vi "RT Driver VI.vi"(7 "Operation":T1, 11 "Device Reference in":T2 format="%.0x") -> (0 "Error Code":i32)   [LabVIEW 2019, in "Telemetry Engine.lvlib"]
uses:
  Telemetry Engine.lvlib
  <vilib>/NI VeriStand/Custom Device API/Custom Device Item Ref.ctl
  <vilib>/NI VeriStand/Custom Device API/Hardware Interface Driver VI Operation.ctl
  Types/Engine State Data.ctl
  Types/Engine Logging Data.ctl
  <vilib>/NI VeriStand/Custom Device API/Block Data Reference.ctl
  <vilib>/NI VeriStand/Custom Device API/Data Reference.ctl
  <vilib>/NI VeriStand/Custom Device API/Global Data Refs.vi
  <vilib>/NI VeriStand/Custom Device API/Custom Device API.lvlib
panel:
  in  "State Data":T3 {"Logging Data"."System Channel Refs" format="%.0x"; "Logging Data"."Block Data Refs"."Data Reference" format="%.0x"}
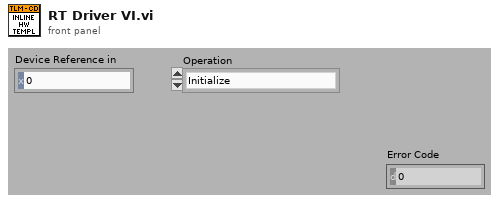
[diagram p1: front panel]
types:
  T1 = typedef "Custom Device API.lvlib/Hardware Interface Driver VI Operation.ctl" = enum16{"Initialize", "Start", "Read Data from HW", "Write Data to HW", "Close"}
  T2 = typedef "Custom Device API.lvlib/Custom Device Item Ref.ctl" = u64
  T3 = typedef "Telemetry Engine.lvlib/Engine State Data.ctl" = cluster{"Data FIFO":refnum<k33>, "Logging Data":T4, "Data FIFO Timeout?":bool, "Data FIFO Timeout Count":dbl, "error":errorcluster}
  T4 = typedef "Telemetry Engine.lvlib/Engine Logging Data.ctl" = cluster{"System Channel Refs":T2[], "Block Data Refs":T5[], "Data Values Array":dbl[], "Data FIFO Timeout Block Ref":i32, "Log File Path":path}
  T5 = typedef "Custom Device API.lvlib/Block Data Reference.ctl" = cluster{"Data Reference":T6, "Offset":u64, "Length":u64}
  T6 = typedef "Custom Device API.lvlib/Data Reference.ctl" = i32
  T7 = cluster{"read mode":enum16{"polling", "blocking"}, "write mode":enum16{"polling", "blocking"}}
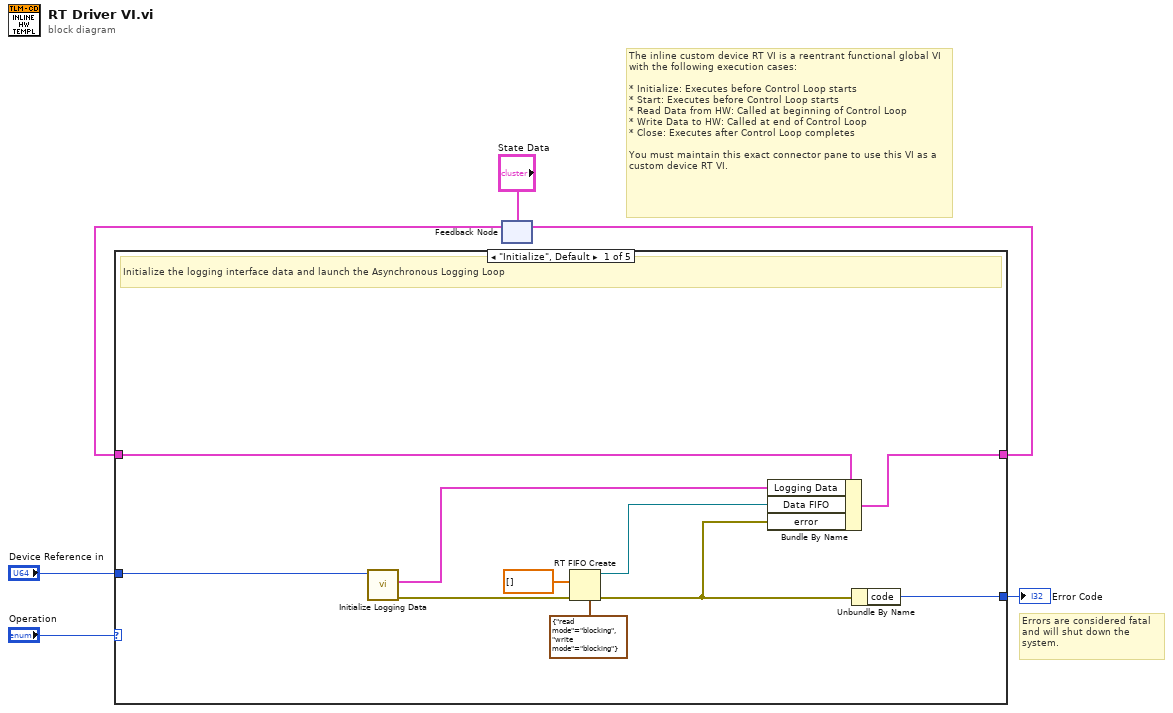
[diagram p0: block diagram]
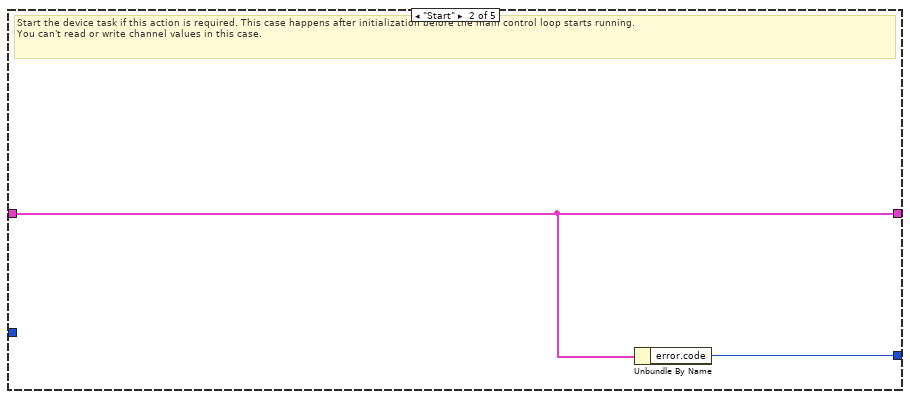
[diagram p2: hidden frame]
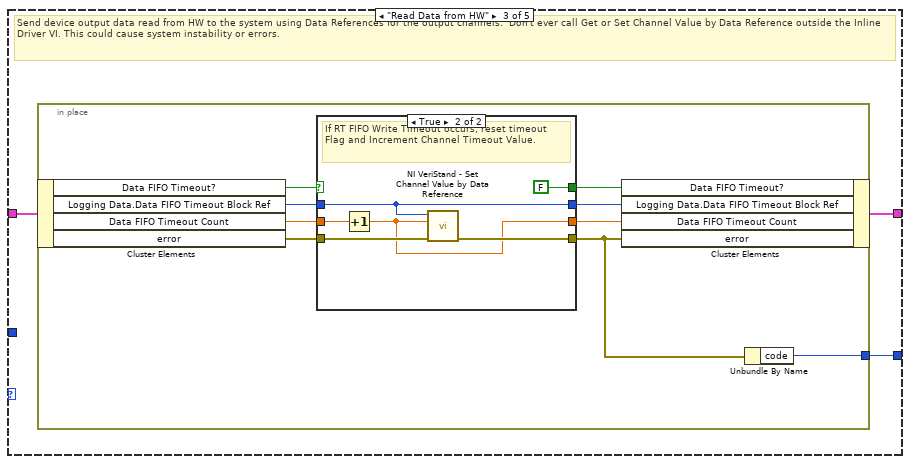
[diagram p3: hidden frame]
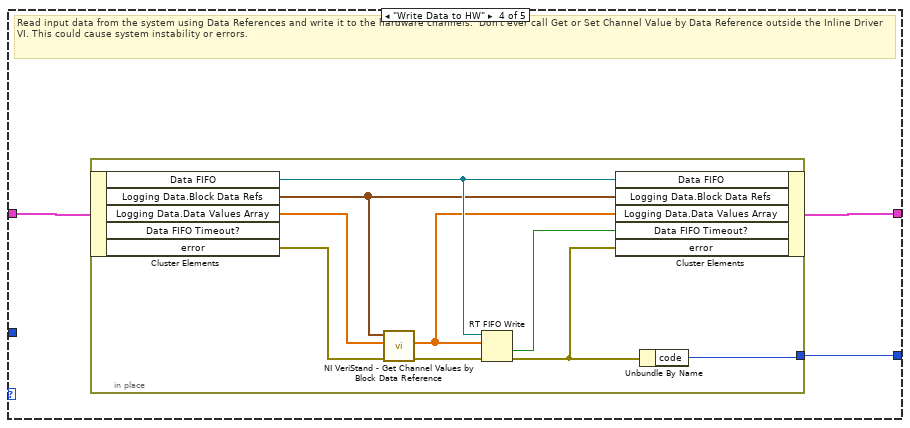
[diagram p5: hidden frame]
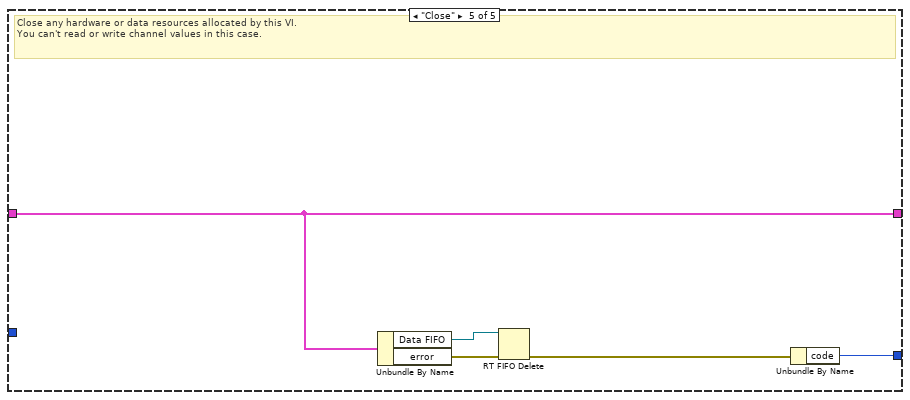
[diagram p6: hidden frame]
diagram:
  # "Errors are considered fatal and will shut down the system."
  # "The inline custom device RT VI is a reentrant functional global VI with the following execution cases:\n\n* Initialize: Executes before Control Loop starts\n* Start: Executes before Control Loop starts\n* Read Data from HW: Called at beginning of Control Loop\n* Write Data to HW: Called at end of Control Loop\n* Close: Executes after Control Loop completes\n\nYou must maintain this exact connector pane to use this VI as a custom device RT VI."
  n1 = feedback #1("State Data") -> (w4:T3)
  n2 = case shown="\"Initialize\", Default" "Operation" {
    tunnel: [w14 w17 w19 w41 w56] -> w5
    tunnel: w4 -> [w13 w17 w20 w42 w56]
    tunnel: "Device Reference in" -> [w9 _ _ _ _]
    tunnel: [w16 w18 w21 w43 w57] -> w2
    frame "Initialize", Default {
      # "Initialize the logging interface data and launch the Asynchronous Logging Loop"
      n3 = call "Initialize Logging Data.vi"("Device Reference in"=w9) -> ("error out"=w7:errorcluster, "Logging Data"=w8:T4)  [unwired: 8 in, 1 out]
      n4 = RT FIFO Create(1:dbl[] [], 3:w7, 7:T7 {"read mode"=enum."blocking", "write mode"=enum."blocking"} ("r/w modes (polling,polling)")) -> (8:w15:refnum<k33>, 11:w12:errorcluster)  [unwired: 5 in, 1 out]
      n5 = Bundle By Name(cluster=w13, "Logging Data"=w8, "Data FIFO"=w15, "error"=w12) -> (w14:T3)
      n6 = Unbundle By Name(w12) -> ("code"=w16:i32)
    }
    frame "Start" {
      # "Start the device task if this action is required. This case happens after initialization before the main control loop starts running.\nYou can't read or write channel values in this case."
      n7 = Unbundle By Name(w17) -> ("error.code"=w18:i32)
    }
    frame "Read Data from HW" {
      # "Send device output data read from HW to the system using Data References for the output channels.  Don't ever call Get or Set Channel Value by Data Reference outside the Inline Driver VI. This could cause system instability or errors."
      n8 = in-place {
        in-place-border: [w30] -> w21
        n9 = in-place-cluster #2(w20) -> ("Data FIFO Timeout?"=w22:bool, "Logging Data.Data FIFO Timeout Block Ref"=w28:i32, "Data FIFO Timeout Count"=w25:dbl, "error"=w26:errorcluster)
        n10 = case shown="True" w22 {
          selector: w22 -> [w34 _]
          tunnel: [w34 FALSE] -> w29
          tunnel: w28 -> [w33 w37]
          tunnel: w26 -> [w32 w39]
          tunnel: [w33 w37] -> w27
          tunnel: [w32 w38] -> w23
          tunnel: w25 -> [w31 w36]
          tunnel: [w31 w35] -> w24
          frame False {
          }
          frame True {
            # "If RT FIFO Write Timeout occurs, reset timeout Flag and Increment Channel Timeout Value."
            n11 = Increment(x=w36) -> (x+1=w35:dbl)
            n12 = call <vilib>:"NI VeriStand - Set Channel Value by Data Reference.vi"("error in (no error)"=w39, "Value"=w35, "Data Reference in"=w37) -> ("error out"=w38:errorcluster)  [unwired: 8 in]
          }
        }
        n13 = in-place-cluster #2("Data FIFO Timeout?"=w29, "Logging Data.Data FIFO Timeout Block Ref"=w27, "Data FIFO Timeout Count"=w24, "error"=w23) -> (w19:T3)
        n14 = Unbundle By Name(w23) -> ("code"=w30:i32)
      }
    }
    frame "Write Data to HW" {
      # "Read input data from the system using Data References and write it to the hardware channels.  Don't ever call Get or Set Channel Value by Data Reference outside the Inline Driver VI. This could cause system instability or errors."
      n15 = in-place {
        in-place-border: [w47] -> w43
        n16 = in-place-cluster #3(w42) -> ("Data FIFO"=w52:refnum<k33>, "Logging Data.Block Data Refs"=w51:T5[], "Logging Data.Data Values Array"=w45:dbl[], "error"=w49:errorcluster)  [unwired: 1 out]
        n17 = call <vilib>:"NI VeriStand - Get Channel Values by Block Data Reference.vi"("error in (no error)"=w49, "Values Array in"=w45, "Block Data Ref"=w51) -> ("error out"=w50:errorcluster, "Values Array out"=w44:dbl[])  [unwired: 6 in, 1 out]
        n18 = RT FIFO Write(0:w52, 1:w44, 3:w50) -> (10:w46:bool, 11:w48:errorcluster)  [unwired: 2 in, 2 out]
        n19 = in-place-cluster #3("Data FIFO"=w52, "Logging Data.Block Data Refs"=w51, "Logging Data.Data Values Array"=w44, "Data FIFO Timeout?"=w46, "error"=w48) -> (w41:T3)
        n20 = Unbundle By Name(w48) -> ("code"=w47:i32)
      }
    }
    frame "Close" {
      # "Close any hardware or data resources allocated by this VI.\nYou can't read or write channel values in this case."
      n21 = Unbundle By Name(w56) -> ("Data FIFO"=w55:refnum<k33>, "error"=w54:errorcluster)
      n22 = RT FIFO Delete(0:w55, 3:w54) -> (11:w53:errorcluster)  [unwired: 1 in]
      n23 = Unbundle By Name(w53) -> ("code"=w57:i32)
    }
  }
  "Error Code" <- w2
  n24 = feedback-in #1(w5) -> ()
